vi "Configure IF Bandwidth.vi"(7 "Enable Reduce IF Bandwidth (T: Enable)":bool=TRUE, 8 "error in (no error)":errorcluster, 9 "Bandwidth (100000 Hz)":dbl=100000.0, 10 "Channel (1)":i32=1, 11 "VISA resource name":refnum<visa-resource-name>) -> (0 "error out":errorcluster, 3 "VISA resource name out":refnum<visa-resource-name>)   [LabVIEW 2018, in "Keysight PNA Series.lvlib"]
doc: "Configures the bandwidth of the digital IF filter."
uses:
  Keysight PNA Series.lvlib
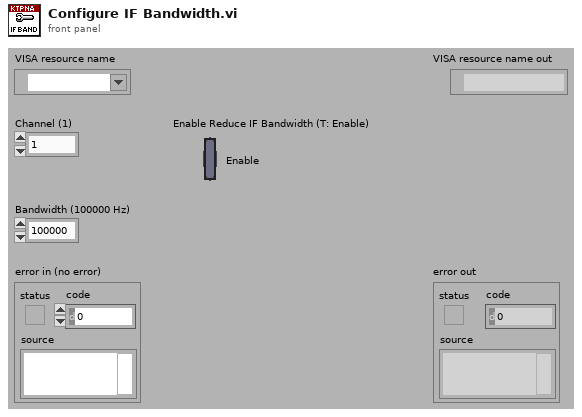
[diagram p1: front panel]
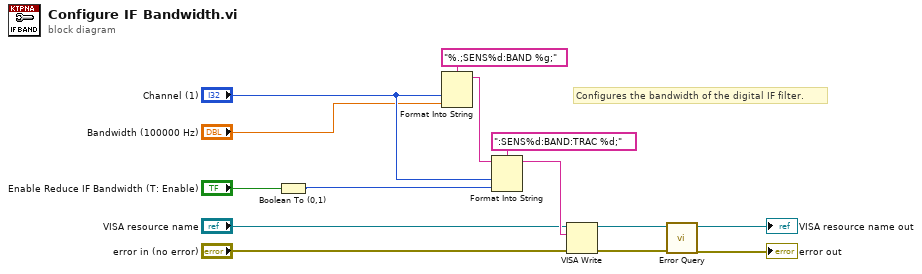
[diagram p0: block diagram]
diagram:
  # "Configures the bandwidth of the digital IF filter."
  n1 = Boolean To (0,1)(Boolean="Enable Reduce IF Bandwidth (T: Enable)") -> (0, 1=w1:i16)
  n2 = Format Into String(format string="%.;SENS%d:BAND %g;", "Channel (1)", "Bandwidth (100000 Hz)") -> (resulting string=w11:string)  [unwired: 2 in, 1 out]
  n3 = Format Into String(format string=":SENS%d:BAND:TRAC %d;", initial string=w11, "Channel (1)", w1) -> (resulting string=w9:string)  [unwired: 1 in, 1 out]
  n4 = VISA Write(VISA resource name="VISA resource name", write buffer=w9, error in (no error)="error in (no error)") -> (VISA resource name out=w6:refnum<visa-resource-name>, error out=w5:errorcluster)  [unwired: 1 out]
  n5 = call "Error Query.vi"("error in (no error)"=w5, "VISA resource name"=w6) -> ("error out"=→"error out":errorcluster, "VISA resource name out"=→"VISA resource name out":refnum<visa-resource-name>)  [unwired: 6 in, 2 out]
